vi "rad_Deploy Images in Parallel.vi"(4 "Deploy":string[](array[string]), 6 "restart after imaging (T)":bool=TRUE, 7 "Deployment Notifiers":T3[](array[typedef]), 8 "error in (no error)":errorcluster, 9 "apply primary NIC from image (F)":bool, 10 "image file path in":path, 11 "Target addresses in":T1[](array[typedef]) {"Primary NIC"."IP Address Request Mode" items=["Static"=1, "DHCP/Link-Local"=2, "Link-Local Only"=4, "DHCP Only"=8]}) -> (0 "Errors Out":errorcluster[](array[cluster]), 2 "image file path out":path, 3 "Target addresses out":T1[](array[typedef]) {"Primary NIC"."IP Address Request Mode" items=["Static"=1, "DHCP/Link-Local"=2, "Link-Local Only"=4, "DHCP Only"=8]})   [LabVIEW 2013]
uses:
  TypeDefs/rad_Deployment Notifiers.ctl
  TypeDefs/rad_Deployment Status Data Type.ctl
  TypeDefs/rad_Deployment Progress Data Type.ctl
  Targets/TypeDefs/rad_Target Information.ctl
  Targets/TypeDefs/rad_Target Network Settings.ctl
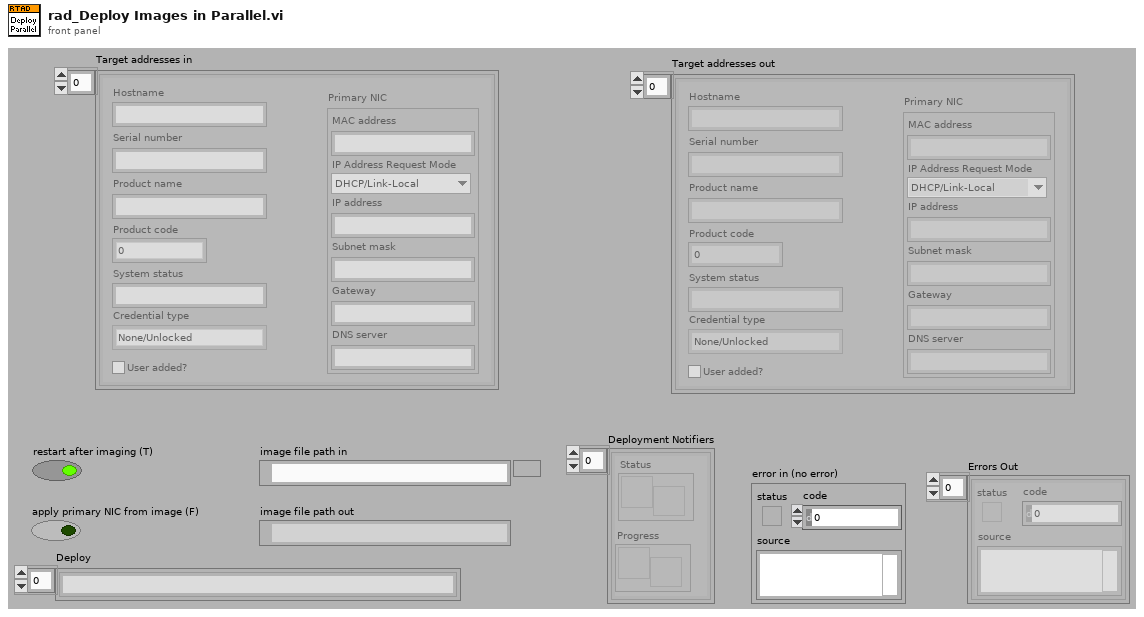
[diagram p1: front panel]
types:
  T1 = typedef "rad_Target Information.ctl" = cluster{"Hostname":string, "Serial number":string, "Product name":string, "Product code":i32, "System status":string, "Credential type":enum16{"None/Unlocked", "FTP Password", "NIAuth Credentials"}, "User added?":bool, "Primary NIC":T2}
  T2 = typedef "rad_Target Network Settings.ctl" = cluster{"MAC address":string, "IP Address Request Mode":i32, "IP address":string, "Subnet mask":string, "Gateway":string, "DNS server":string}
  T3 = typedef "rad_Deployment Notifiers.ctl" = cluster{"Status":refnum<notifier>, "Progress":refnum<notifier>}
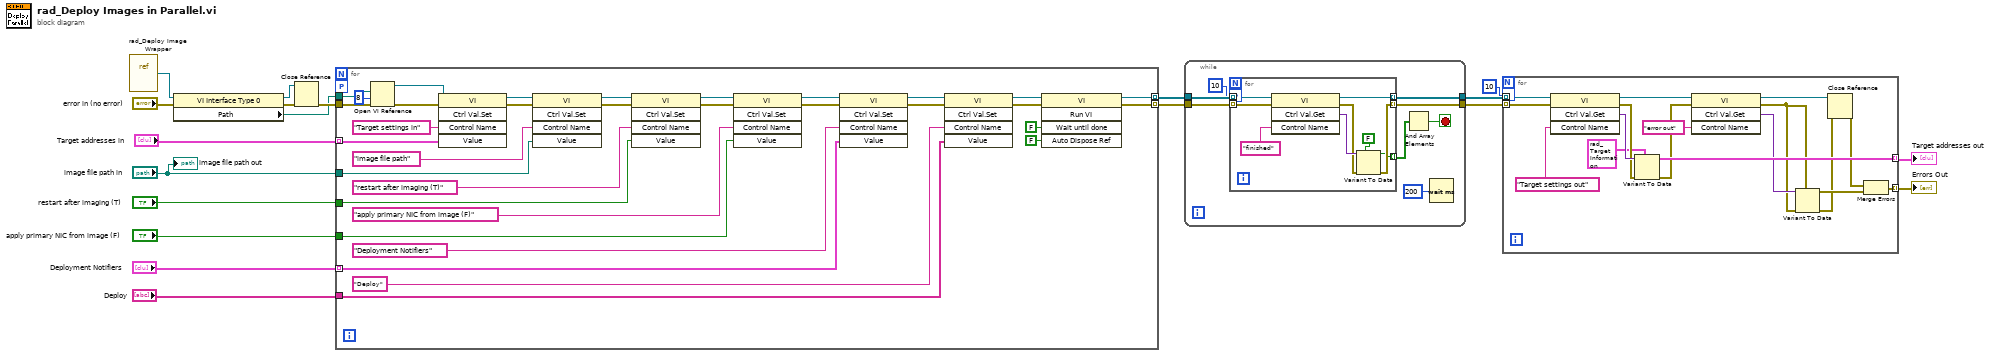
[diagram p0: block diagram]
diagram:
  n1 = vi-ref "rad_Deploy Image Wrapper.vi"() -> (w19:refnum<vi>)
  n2 = property class="VI Interface Type 0"(reference=w19, error in="error in (no error)") -> (reference out=w18:refnum<vi>, error out=w17:errorcluster, "Path"=w15:path)
  n3 = Close Reference(reference=w18, error in (no error)=w17) -> (error out=w16:errorcluster)
  n4 = for {
    tunnel: w16 -> [w52]
    tunnel: w15 -> [w51]
    tunnel: "Target addresses in" -> [w47] mode=indexing
    tunnel: "image file path in" -> [w43]
    tunnel: "restart after imaging (T)" -> [w39]
    tunnel: [w36] -> w12 mode=indexing
    tunnel: [w35] -> w11 mode=indexing
    tunnel: "apply primary NIC from image (F)" -> [w30]
    tunnel: "Deployment Notifiers" -> [w27] mode=indexing
    tunnel: "Deploy" -> [w23]
    workers-P: _ -> [_]
    n5 = Open VI Reference(vi path=w51, options=8, error in (no error)=w52) -> (vi reference=w50:refnum<vi>, error out=w49:errorcluster)  [unwired: 3 in]
    n6 = invoke class="VI" method="Ctrl Val.Set"(reference=w50, error in=w49, "Control Name"="Target settings in", "Value"=w47) -> (reference out=w46:refnum<vi>, error out=w45:errorcluster)  [unwired: 1 in, 3 out]
    n7 = invoke class="VI" method="Ctrl Val.Set"(reference=w46, error in=w45, "Control Name"="image file path", "Value"=w43) -> (reference out=w42:refnum<vi>, error out=w41:errorcluster)  [unwired: 1 in, 3 out]
    n8 = invoke class="VI" method="Ctrl Val.Set"(reference=w42, error in=w41, "Control Name"="restart after imaging (T)", "Value"=w39) -> (reference out=w33:refnum<vi>, error out=w32:errorcluster)  [unwired: 1 in, 3 out]
    n9 = invoke class="VI" method="Ctrl Val.Set"(reference=w33, error in=w32, "Control Name"="apply primary NIC from image (F)", "Value"=w30) -> (reference out=w29:refnum<vi>, error out=w28:errorcluster)  [unwired: 1 in, 3 out]
    n10 = invoke class="VI" method="Ctrl Val.Set"(reference=w29, error in=w28, "Control Name"="Deployment Notifiers", "Value"=w27) -> (reference out=w21:refnum<vi>, error out=w22:errorcluster)  [unwired: 1 in, 3 out]
    n11 = invoke class="VI" method="Ctrl Val.Set"(reference=w21, error in=w22, "Control Name"="Deploy", "Value"=w23) -> (reference out=w26:refnum<vi>, error out=w25:errorcluster)  [unwired: 1 in, 3 out]
    n12 = invoke class="VI" method="Run VI"(reference=w26, error in=w25, "Wait until done"=FALSE ("Wait Until Done"), "Auto Dispose Ref"=FALSE ("Auto Dispose Reference")) -> (reference out=w36:refnum<vi>, error out=w35:errorcluster)  [unwired: 1 in, 3 out]
  }
  n13 = while {
    tunnel: w12 -> [w58]
    tunnel: w11 -> [w57]
    tunnel: [w55] -> w9
    tunnel: [w56] -> w10
    stop <- w59 stop-if-true
    n14 = for {
      tunnel: w58 -> [w69] mode=indexing
      tunnel: w57 -> [w68] mode=indexing
      tunnel: [w66] -> w56 mode=indexing
      tunnel: [w62] -> w55 mode=indexing
      tunnel: [w61] -> w54 mode=indexing
      workers-P: 10 -> [_]
      n15 = invoke class="VI" method="Ctrl Val.Get"(reference=w69, error in=w68, "Control Name"="finished") -> (reference out=w66:refnum<vi>, error out=w63:errorcluster, "Get Control Value Variant"=w64:variant)  [unwired: 1 in, 1 out]
      n16 = Variant To Data(error in=w63, type=FALSE, Variant=w64) -> (data=w61:bool, error out=w62:errorcluster)
    }
    n17 = And Array Elements(Boolean array=w54) -> (logical AND=w59:bool)
    n18 = Wait (ms)(milliseconds to wait=u32 200) -> ()  [unwired: 1 out]
  }
  n19 = for {
    tunnel: w10 -> [w86] mode=indexing
    tunnel: w9 -> [w85] mode=indexing
    tunnel: [w82] -> w1 mode=indexing
    tunnel: [w74] -> w8 mode=indexing
    workers-P: 10 -> [_]
    n20 = invoke class="VI" method="Ctrl Val.Get"(reference=w86, error in=w85, "Control Name"="Target settings out") -> (reference out=w81:refnum<vi>, error out=w80:errorcluster, "Get Control Value Variant"=w83:variant)  [unwired: 1 in, 1 out]
    n21 = Variant To Data(error in=w80, type=T1 {"Hostname"="", "Serial number"="", "Product name"="", "Product code"=0, "System status"="", "Credential type"=enum."None/Unlocked", "User added?"=FALSE, "Primary NIC"={"MAC address"="", "IP Address Request Mode"=0, "IP address"="", "Subnet mask"="", "Gateway"="", "DNS server"=""}} ("Target settings"), Variant=w83) -> (data=w82:T1, error out=w79:errorcluster)
    n22 = invoke class="VI" method="Ctrl Val.Get"(reference=w81, error in=w79, "Control Name"="error out") -> (reference out=w73:refnum<vi>, error out=w76:errorcluster, "Get Control Value Variant"=w77:variant)  [unwired: 1 in, 1 out]
    n23 = Variant To Data(error in=w76, type=w76, Variant=w77) -> (data=w75:errorcluster, error out=w72:errorcluster)
    n24 = Close Reference(reference=w73, error in (no error)=w72) -> (error out=w71:errorcluster)
    n25 = Merge Errors(w71, w75) -> (w74:errorcluster)
  }
  "Errors Out" <- w8
  "Target addresses out" <- w1
  "image file path out" <- "image file path in"
